vi "Elapsed Time.vi"() -> (2 "Elapsed Time":u32)   [LabVIEW 2014, in "Endigit.lvlib"]
uses:
  Endigit.lvlib
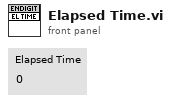
[diagram p1: front panel]
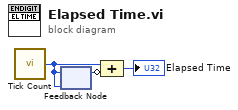
[diagram p0: block diagram]
diagram:
  n1 = call "Tick Count"() -> ("Tick Count(mSec)"=w2:u32)
  n2 = feedback-in #1(w2) -> ()
  n3 = feedback #1(w2) -> (w3:u32)
  n4 = Compound Arithmetic op=ADD(w2, invert w3) -> (→"Elapsed Time":u32)
